vi "get_threading.vi"(8 "error in (no error)":errorcluster, 11 "system in":refnum<class "system.lvclass">) -> (0 "error out":errorcluster, 2 "system.threading.lvclass":refnum<class "system.threading.lvclass">, 3 "system out":refnum<class "system.lvclass">)   [LabVIEW 2021, in "system.lvclass"]
uses:
  system.lvclass
  system.lvclass/system.ctl
  system.threading/system.threading.lvclass
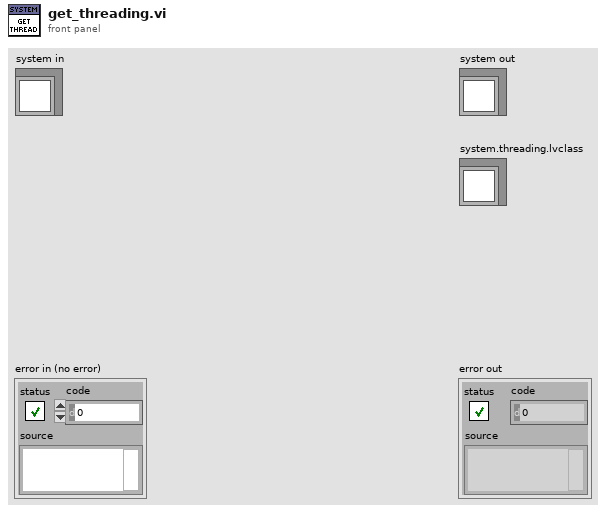
[diagram p1: front panel]
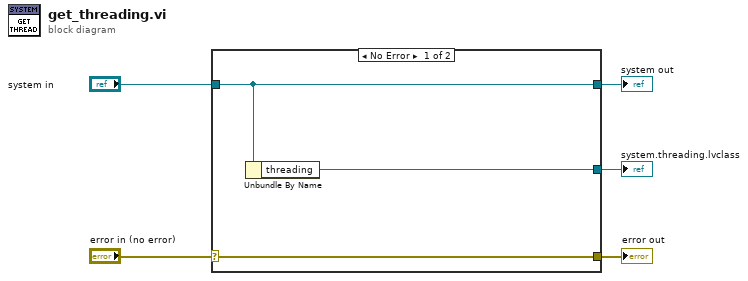
[diagram p0: block diagram]
diagram:
  n1 = case shown="No Error" "error in (no error)" {
    selector: "error in (no error)" -> [w8 w9]
    tunnel: [w8 w9] -> w4
    tunnel: [w7 w10] -> w2
    tunnel: "system in" -> [w7 w10]
    tunnel: [w6 _] -> w1
    frame No Error {
      n2 = Unbundle By Name(w7) -> ("threading"=w6:refnum<class "system.threading.lvclass">)
    }
    frame Error {
    }
  }
  "error out" <- w4
  "system out" <- w2
  "system.threading.lvclass" <- w1
